vi "Begin.vi"(11 "Image Size":T3=enum."160x120") -> (0 "error out":errorcluster)   [LabVIEW 2012]
doc: "Called before other user functions, this VI is expected to open initial I/O refnums, load in file data, and do all program initialization. Notice that the <B>error out</B> terminal is simply used for data flow. Wiring it to other structures or subVIs ensures that this VI runs first."
uses:
  <vilib>/Rock Robotics/WPI/Camera/WPI_CameraImageSize.ctl
  <vilib>/Rock Robotics/SystemInterfaces/DIO/FPGA_DIOChannel.ctl
  <vilib>/Rock Robotics/SystemInterfaces/Typedef/FPGA_TypedefDigitalModule.ctl
  <vilib>/Rock Robotics/WPI/Joystick/WPI_JoystickDeviceEnum.ctl
  <vilib>/Rock Robotics/WPI/Camera/WPI_CameraWhite Balance Values.ctl
  <vilib>/Rock Robotics/WPI/Camera/WPI_CameraExposure Values.ctl
  <vilib>/Rock Robotics/WPI/Camera/WPI_CameraFrameRate.ctl
  <vilib>/Rock Robotics/SystemInterfaces/DIO/FPGA_DIOPWMChannel.ctl
  <vilib>/Rock Robotics/SystemInterfaces/AI/FPGA_AIChannel.ctl
  <vilib>/Rock Robotics/WPI/Encoder/WPI_EncoderType.ctl
  <vilib>/Rock Robotics/WPI/RobotDrive/WPI_RobotDriveOpen2MotorWithVictor.vi
  <vilib>/Rock Robotics/WPI/Counter/WPI_CounterDigitalInputToDigitalSource.vi
  <vilib>/Rock Robotics/WPI/MotorControl/WPI_MotorControlOpen Victor.vi
panel:
  in  "DIO Module 4":T1
  in  "B Channel 4":T2=enum."DIO 7"
  in  "A Channel 4":T2=enum."DIO 6"
  in  "DIO Module 3":T1
  in  "B Channel 3":T2=enum."DIO 5"
  in  "A Channel 3":T2=enum."DIO 4"
  in  "DIO Module 2":T1
  in  "B Channel 2":T2=enum."DIO 9"
  in  "A Channel 2":T2=enum."DIO 8"
  in  "DIO Module":T1
  in  "B Channel":T2=enum."DIO 12"
  in  "A Channel":T2=enum."DIO 11"
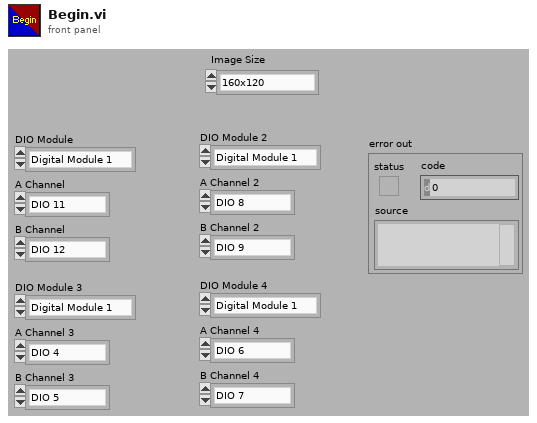
[diagram p1: front panel]
types:
  T1 = typedef "FPGA_TypedefDigitalModule.ctl" = enum16{"Digital Module 1", "Digital Module 2"}
  T2 = typedef "FPGA_DIOChannel.ctl" = enum8{"DIO 1", "DIO 2", "DIO 3", "DIO 4", "DIO 5", "DIO 6", "DIO 7", "DIO 8", "DIO 9", "DIO 10", "DIO 11", "DIO 12", "DIO 13", "DIO 14", "Invalid"}
  T3 = typedef "WPI_CameraImageSize.ctl" = enum16{"640x480", "320x240", "160x120"}
  T4 = typedef "WPI_EncoderType.ctl" = enum16{"1x", "2x", "4x"}
  T5 = typedef "FPGA_DIOPWMChannel.ctl" = enum8{"PWM 1", "PWM 2", "PWM 3", "PWM 4", "PWM 5", "PWM 6", "PWM 7", "PWM 8", "PWM 9", "PWM 10", "Invalid"}
  T6 = typedef "FPGA_AIChannel.ctl" = enum8{"AI 1", "AI 2", "AI 3", "AI 4", "AI 5", "AI 6", "AI 7", "AI 8", "Invalid"}
  T7 = typedef "WPI_CameraFrameRate.ctl" = u32
  T8 = typedef "WPI_CameraExposure Values.ctl" = enum16{"Auto", "Flicker-free 50 Hz", "Flicker-free 60 Hz", "Hold current"}
  T9 = typedef "WPI_CameraWhite Balance Values.ctl" = enum16{"Auto", "Fixed indoor", "Fixed outdoor 1", "Fixed outdoor 2", "Fixed fluorescent 1", "Fixed fluorescent 2", "Hold current"}
  T10 = typedef "WPI_JoystickDeviceEnum.ctl" = enum16{"USB 1", "USB 2", "USB 3", "USB 4", "Kinect 1", "Kinect 2"}
  T11 = typedef "WPI_DigitalInputDevRef.ctl" = cluster{"DevStatus":errorcluster, "DIO Channel":T2, "Digital Module":T1}
  T12 = typedef "FPGA_CounterEncoderSourceConvertionLVSourceType.ctl" = cluster{"DevStatus":errorcluster, "AnalogTriggerMode?":bool, "DigitalMode":cluster{"Digital Module":T1, "DIO Channel":T13}, "AnalogTriggerMode":cluster{"AnalogTriggerIndex":T14, "OutputType":T15}}
  T13 = typedef "FPGA_DIODigitalSourceChannel.ctl" = enum8{"DIO 1", "DIO 2", "DIO 3", "DIO 4", "DIO 5", "DIO 6", "DIO 7", "DIO 8", "DIO 9", "DIO 10", "DIO 11", "DIO 12", "DIO 13", "DIO 14", "Disabled"}
  T14 = typedef "FPGA_AnalogTriggerIndex.ctl" = enum8{"Trig 0", "Trig 1", "Trig 2", "Trig 3", "Trig 4", "Trig 5", "Trig 6", "Trig 7", "Invalid"}
  T15 = typedef "FPGA_AnalogTriggerOutType.ctl" = enum16{"InWindow", "TriggerState", "Rising", "Falling"}
  T16 = typedef "WPI_JoystickDevRef.ctl" = cluster{"Device":T10}
  T17 = typedef "WPI_CameraDevRef.ctl" = cluster{"Camera Address":string, "CameraStatus":errorcluster, "Acquire Image Notifier":refnum<notifier>}
  T18 = typedef "WPI_RobotDriveDevRef.ctl" = cluster{"DevStatus":errorcluster, "Motors[]":T19[], "Square Inputs":bool, "Max Output":dbl, "Isochronous":bool}
  T19 = typedef "WPI_MotorControlDeviceRef.ctl" = cluster{"DeviceStatus":errorcluster, "Type":enum16{"PWM", "CAN"}, "PWM":cluster{"Digital Module":T1, "PWM Channel":T5, "DeadBand":T20}, "CAN":cluster{"Device Number":u8, "Control Mode":T21, "Semaphore":T22, "Max Vout":dbl}, "Invert":bool, "TransformRef":T23, "InvTransformRef":T23}
  T20 = typedef "WPI_PWMDeadband.ctl" = cluster{"Name":string, "maxPositivePwm":i32, "minPositivePwm":i32, "centerPwm":i32, "maxNegativePwm":i32, "minNegativePwm":i32, "angularRange":u16}
  T21 = typedef "WPI_CANJaguar_ControlMode.ctl" = enum8{"Percent VBus", "Current", "Speed", "Position", "Voltage"}
  T22 = typedef "Semaphore RefNum" = refnum<k1>
  T23 = typedef "WPI_PWMTransform_ConPane.ctl" = refnum<vi>
  T24 = typedef "WPI_EncoderDevRef.ctl" = cluster{"DevStatus":errorcluster, "EncoderIndex":T25, "CounterIndex":T26, "DistancePerCount":dbl, "Decoding Type":T4}
  T25 = typedef "FPGA_EncoderIdx.ctl" = enum8{"Enc 0", "Enc 1", "Enc 2", "Enc 3", "Invalid"}
  T26 = typedef "FPGA_CounterCtrSystemIndex.ctl" = enum8{"Ctr 0", "Ctr 1", "Ctr 2", "Ctr 3", "Ctr 4", "Ctr 5", "Ctr 6", "Ctr 7", "Invalid"}
  T27 = typedef "WPI_AnalogChannelDevRef.ctl" = cluster{"DevStatus":errorcluster, "Analog Module":T28, "Analog Channel":T6}
  T28 = typedef "FPGA_TypedefAnalogModule.ctl" = enum16{"Analog Module 1", "Analog Module 2"}
  T29 = typedef "WPI_DigitalOutputDevRef.ctl" = cluster{"Digital Module":T1, "DIO Channel":T2, "DevStatus":errorcluster}
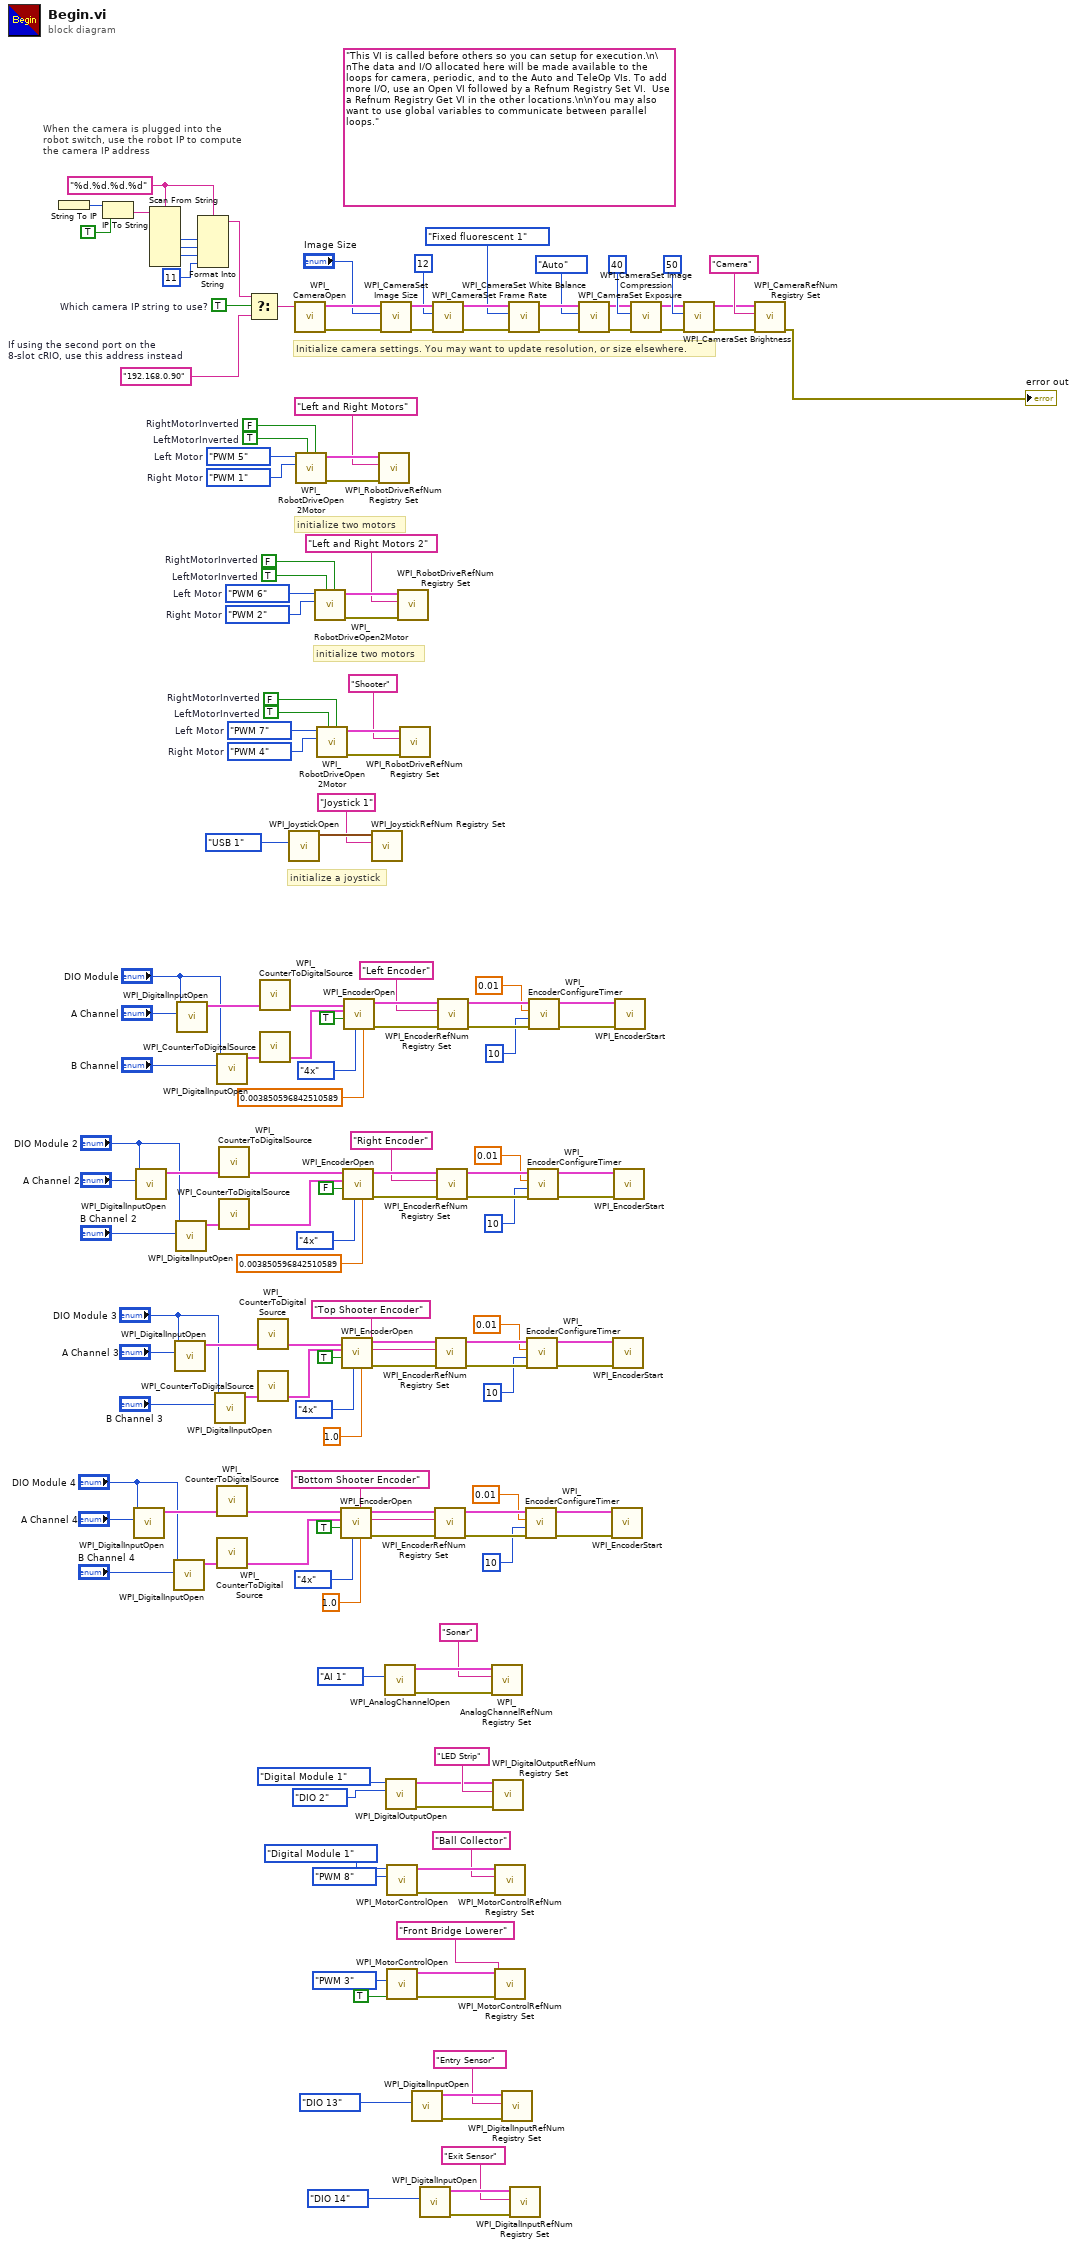
[diagram p0: block diagram]
diagram:
  w95 = FPGA_DIOPWMChannel."PWM 1"  # Right Motor
  w96 = FPGA_DIOPWMChannel."PWM 5"  # Left Motor
  w100 = TRUE  # LeftMotorInverted
  w101 = FALSE  # RightMotorInverted
  w102 = FPGA_DIOPWMChannel."PWM 2"  # Right Motor
  w103 = FPGA_DIOPWMChannel."PWM 6"  # Left Motor
  w107 = TRUE  # LeftMotorInverted
  w108 = FALSE  # RightMotorInverted
  w119 = FPGA_DIOPWMChannel."PWM 4"  # Right Motor
  w120 = FPGA_DIOPWMChannel."PWM 7"  # Left Motor
  w124 = TRUE  # LeftMotorInverted
  w125 = FALSE  # RightMotorInverted
  w126 = TRUE  # Which camera IP string to use?
  w130 = "%d.%d.%d.%d" ("format string")
  (unwired) "This VI is called before others so you can setup for execution.\n\nThe data and I/O allocated here will be made available to the loops for camera, periodic, and to the Auto and TeleOp VIs. To add more I/O, use an Open VI followed by a Refnum Registry Set VI.  Use a Refnum Registry Get VI in the other locations.\n\nYou may also want to use global variables to communicate between parallel loops."
  w127 = "192.168.0.90"  # If using the second port on the 8-slot cRIO, use this address instead
  # "initialize two motors"
  # "initialize two motors"
  # "When the camera is plugged into the\nrobot switch, use the robot IP to compute\nthe camera IP address"
  # "initialize a joystick"
  # "Initialize camera settings. You may want to update resolution, or size elsewhere."
  n1 = String To IP() -> (0:w137:u32)  [unwired: 1 in]
  n2 = IP To String(1:TRUE ("dot notation? (F)"), 2:w137) -> (0:w135:string)
  n3 = call <vilib>:"WPI_DigitalInputOpen.vi"("DIO Channel"="A Channel 4", "Digital Module (Module 1)"="DIO Module 4") -> ("DigitalInputDevRef"=w9:T11)  [unwired: 1 in, 8 out]
  n4 = call <vilib>:"WPI_DigitalInputOpen.vi"("DIO Channel"="A Channel 2", "Digital Module (Module 1)"="DIO Module 2") -> ("DigitalInputDevRef"=w69:T11)  [unwired: 1 in, 8 out]
  n5 = Scan From String(format string=w130, input string=w135) -> (output 1=w134:i32, output 2=w133:i32, output 3=w132:i32)  [unwired: 7 in, 3 out]
  n6 = call <vilib>:"WPI_DigitalInputOpen.vi"("DIO Channel"="B Channel 4", "Digital Module (Module 1)"="DIO Module 4") -> ("DigitalInputDevRef"=w10:T11)  [unwired: 1 in, 8 out]
  n7 = call <vilib>:"WPI_DigitalInputOpen.vi"("DIO Channel"="A Channel 3", "Digital Module (Module 1)"="DIO Module 3") -> ("DigitalInputDevRef"=w16:T11)  [unwired: 1 in, 8 out]
  n8 = call <vilib>:"WPI_DigitalInputOpen.vi"("DIO Channel"="B Channel 2", "Digital Module (Module 1)"="DIO Module 2") -> ("DigitalInputDevRef"=w70:T11)  [unwired: 1 in, 8 out]
  n9 = call <vilib>:"WPI_DigitalInputOpen.vi"("DIO Channel"="A Channel", "Digital Module (Module 1)"="DIO Module") -> ("DigitalInputDevRef"=w76:T11)  [unwired: 1 in, 8 out]
  n10 = Format Into String(format string=w130, w134, w133, w132, 11 ("Compression")) -> (resulting string=w128:string)  [unwired: 2 in, 1 out]
  n11 = call <vilib>:"WPI_DigitalInputOpen.vi"("DIO Channel"="B Channel 3", "Digital Module (Module 1)"="DIO Module 3") -> ("DigitalInputDevRef"=w17:T11)  [unwired: 1 in, 8 out]
  n12 = call <vilib>:"WPI_DigitalInputOpen.vi"("DIO Channel"="B Channel", "Digital Module (Module 1)"="DIO Module") -> ("DigitalInputDevRef"=w77:T11)  [unwired: 1 in, 8 out]
  n13 = call-poly <vilib>:"WPI_CounterToDigitalSource.vi"("DigitalInputDevRef"=w9) -> ("Digital Source"=w4:T12)  [unwired: 6 out]
  n14 = call-poly <vilib>:"WPI_CounterToDigitalSource.vi"("DigitalInputDevRef"=w10) -> ("Digital Source"=w5:T12)  [unwired: 6 out]
  n15 = call-poly <vilib>:"WPI_CounterToDigitalSource.vi"("DigitalInputDevRef"=w69) -> ("Digital Source"=w64:T12)  [unwired: 6 out]
  n16 = call-poly <vilib>:"WPI_CounterToDigitalSource.vi"("DigitalInputDevRef"=w70) -> ("Digital Source"=w65:T12)  [unwired: 6 out]
  n17 = Select(t=w128, s=w126, f=w127) -> (s? t:f=w129:string)
  n18 = call-poly <vilib>:"WPI_CounterToDigitalSource.vi"("DigitalInputDevRef"=w16) -> ("Digital Source"=w11:T12)  [unwired: 6 out]
  n19 = call-poly <vilib>:"WPI_CounterToDigitalSource.vi"("DigitalInputDevRef"=w17) -> ("Digital Source"=w12:T12)  [unwired: 6 out]
  n20 = call-poly <vilib>:"WPI_CounterToDigitalSource.vi"("DigitalInputDevRef"=w76) -> ("Digital Source"=w71:T12)  [unwired: 6 out]
  n21 = call-poly <vilib>:"WPI_CounterToDigitalSource.vi"("DigitalInputDevRef"=w77) -> ("Digital Source"=w72:T12)  [unwired: 6 out]
  n22 = call <vilib>:"WPI_JoystickOpen.vi"("JoystickDevice"=WPI_JoystickDeviceEnum."USB 1") -> ("JoystickDevRef"=w160:T16)  [unwired: 10 out]
  n23 = call <vilib>:"WPI_CameraOpen.vi"("Camera Address"=w129) -> ("error out"=w150:errorcluster, "CameraDevRef"=w151:T17)  [unwired: 2 in, 7 out]
  n24 = call-poly <vilib>:"WPI_RobotDriveOpen2Motor.vi"("Right Motor Inverted"=w101, "Left Motor Inverted"=w100, "Right Motor"=w95, "Left Motor"=w96) -> ("error out"=w97:errorcluster, "RobotDriveDevRef"=w99:T18)  [unwired: 1 in, 5 out]
  n25 = call-poly <vilib>:"WPI_RobotDriveOpen2Motor.vi"("Right Motor Inverted"=w108, "Left Motor Inverted"=w107, "Right Motor"=w102, "Left Motor"=w103) -> ("error out"=w104:errorcluster, "RobotDriveDevRef"=w106:T18)  [unwired: 1 in, 5 out]
  n26 = call-poly <vilib>:"WPI_RobotDriveOpen2Motor.vi"("Right Motor Inverted"=w125, "Left Motor Inverted"=w124, "Right Motor"=w119, "Left Motor"=w120) -> ("error out"=w121:errorcluster, "RobotDriveDevRef"=w123:T18)  [unwired: 1 in, 5 out]
  n27 = call <vilib>:"WPI_EncoderOpen.vi"("DistancePerCount"=1.0, "Decoding Type"=WPI_EncoderType."4x", "Invert Direction (False)"=TRUE, "BSource"=w5, "ASource"=w4) -> ("error out"=w25:errorcluster, "EncoderDevRef"=w26:T24)  [unwired: 5 in]
  n28 = call <vilib>:"WPI_EncoderOpen.vi"("DistancePerCount"=1.0, "Decoding Type"=WPI_EncoderType."4x", "Invert Direction (False)"=TRUE, "BSource"=w12, "ASource"=w11) -> ("error out"=w36:errorcluster, "EncoderDevRef"=w37:T24)  [unwired: 5 in]
  n29 = call <vilib>:"WPI_EncoderOpen.vi"("DistancePerCount"=0.003850596842510589, "Decoding Type"=WPI_EncoderType."4x", "Invert Direction (False)"=FALSE, "BSource"=w65, "ASource"=w64) -> ("error out"=w85:errorcluster, "EncoderDevRef"=w86:T24)  [unwired: 5 in]
  n30 = call <vilib>:"WPI_EncoderOpen.vi"("DistancePerCount"=0.003850596842510589, "Decoding Type"=WPI_EncoderType."4x", "Invert Direction (False)"=TRUE, "BSource"=w72, "ASource"=w71) -> ("error out"=w111:errorcluster, "EncoderDevRef"=w112:T24)  [unwired: 5 in]
  n31 = call <vilib>:"WPI_JoystickRefNum Registry Set.vi"("refnum name"="Joystick 1", "JoystickDevRef"=w160) -> ()  [unwired: 1 in, 9 out]
  n32 = call <vilib>:"WPI_RobotDriveRefNum Registry Set.vi"("error in (no error)"=w97, "refnum name"="Left and Right Motors", "RobotDriveDevRef"=w99) -> ()  [unwired: 9 out]
  n33 = call <vilib>:"WPI_CameraSet Image Size.vi"("error in (no error)"=w150, "Image Size"="Image Size", "CameraDevRef"=w151) -> ("error out"=w149:errorcluster, "CameraDevRef Out"=w152:T17)  [unwired: 7 out]
  n34 = call <vilib>:"WPI_AnalogChannelOpen.vi"("Analog Channel"=FPGA_AIChannel."AI 1") -> ("error out"=w116:errorcluster, "AIDeviceRef"=w118:T27)  [unwired: 9 in]
  n35 = call <vilib>:"WPI_DigitalOutputOpen.vi"("DIO Channel"=FPGA_DIOChannel."DIO 2", "Digital Module (Module 1)"=FPGA_TypedefDigitalModule."Digital Module 1") -> ("error out"=w44:errorcluster, "DigitalOutputDevRef"=w45:T29)  [unwired: 8 in]
  n36 = call-poly <vilib>:"WPI_MotorControlOpen.vi"("PWM Channel"=FPGA_DIOPWMChannel."PWM 8", "Digital Module (Module 1)"=FPGA_TypedefDigitalModule."Digital Module 1") -> ("error out"=w62:errorcluster, "MotorControlDeviceRef"=w61:T19)  [unwired: 8 in]
  n37 = call-poly <vilib>:"WPI_MotorControlOpen.vi"("Invert"=TRUE, "PWM Channel"=FPGA_DIOPWMChannel."PWM 3") -> ("error out"=w58:errorcluster, "MotorControlDeviceRef"=w57:T19)  [unwired: 8 in]
  n38 = call <vilib>:"WPI_RobotDriveRefNum Registry Set.vi"("error in (no error)"=w104, "refnum name"="Left and Right Motors 2", "RobotDriveDevRef"=w106) -> ()  [unwired: 9 out]
  n39 = call <vilib>:"WPI_RobotDriveRefNum Registry Set.vi"("error in (no error)"=w121, "refnum name"="Shooter", "RobotDriveDevRef"=w123) -> ()  [unwired: 9 out]
  n40 = call <vilib>:"WPI_DigitalInputOpen.vi"("DIO Channel"=FPGA_DIOChannel."DIO 13") -> ("error out"=w54:errorcluster, "DigitalInputDevRef"=w55:T11)  [unwired: 9 in]
  n41 = call <vilib>:"WPI_DigitalInputOpen.vi"("DIO Channel"=FPGA_DIOChannel."DIO 14") -> ("error out"=w50:errorcluster, "DigitalInputDevRef"=w51:T11)  [unwired: 9 in]
  n42 = call <vilib>:"WPI_CameraSet Frame Rate.vi"("error in (no error)"=w149, "Frame Rate (fps)"=T7 12, "CameraDevRef"=w152) -> ("error out"=w148:errorcluster, "CameraDevRef Out"=w154:T17)  [unwired: 7 out]
  n43 = call <vilib>:"WPI_EncoderRefNum Registry Set.vi"("error in (no error)"=w25, "refnum name"="Bottom Shooter Encoder", "EncoderDevRef"=w26) -> ("error out"=w21:errorcluster, "EncoderDevRef"=w23:T24)  [unwired: 7 in]
  n44 = call <vilib>:"WPI_EncoderRefNum Registry Set.vi"("error in (no error)"=w36, "refnum name"="Top Shooter Encoder", "EncoderDevRef"=w37) -> ("error out"=w32:errorcluster, "EncoderDevRef"=w34:T24)  [unwired: 7 in]
  n45 = call <vilib>:"WPI_EncoderRefNum Registry Set.vi"("error in (no error)"=w85, "refnum name"="Right Encoder", "EncoderDevRef"=w86) -> ("error out"=w81:errorcluster, "EncoderDevRef"=w83:T24)  [unwired: 7 in]
  n46 = call <vilib>:"WPI_EncoderRefNum Registry Set.vi"("error in (no error)"=w111, "refnum name"="Left Encoder", "EncoderDevRef"=w112) -> ("error out"=w92:errorcluster, "EncoderDevRef"=w94:T24)  [unwired: 7 in]
  n47 = call <vilib>:"WPI_AnalogChannelRefNum Registry Set.vi"("error in (no error)"=w116, "refnum name"="Sonar", "AIDeviceRef"=w118) -> ()  [unwired: 7 in, 2 out]
  n48 = call <vilib>:"WPI_DigitalOutputRefNum Registry Set.vi"("error in (no error)"=w44, "refnum name"="LED Strip", "DigitalOutputDevRef"=w45) -> ()  [unwired: 7 in, 2 out]
  n49 = call <vilib>:"WPI_MotorControlRefNum Registry Set.vi"("error in (no error)"=w62, "refnum name"="Ball Collector", "MotorControlDevRef"=w61) -> ()  [unwired: 7 in, 2 out]
  n50 = call <vilib>:"WPI_MotorControlRefNum Registry Set.vi"("error in (no error)"=w58, "refnum name"="Front Bridge Lowerer", "MotorControlDevRef"=w57) -> ()  [unwired: 7 in, 2 out]
  n51 = call <vilib>:"WPI_DigitalInputRefNum Registry Set.vi"("error in (no error)"=w54, "refnum name"="Entry Sensor", "DigitalInputDevRef"=w55) -> ()  [unwired: 7 in, 2 out]
  n52 = call <vilib>:"WPI_CameraSet White Balance.vi"("error in (no error)"=w148, "White Balance"=WPI_CameraWhite_Balance_Values."Fixed fluorescent 1", "CameraDevRef"=w154) -> ("error out"=w147:errorcluster, "CameraDevRef Out"=w153:T17)  [unwired: 7 out]
  n53 = call <vilib>:"WPI_DigitalInputRefNum Registry Set.vi"("error in (no error)"=w50, "refnum name"="Exit Sensor", "DigitalInputDevRef"=w51) -> ()  [unwired: 7 in, 2 out]
  n54 = call <vilib>:"WPI_EncoderConfigureTimer.vi"("error in (no error)"=w21, "Number Samples to Average"=u8 10, "Minimum Rate"=0.01, "EncoderDevRef"=w23) -> ("error out"=w20:errorcluster, "EncoderDevRef"=w22:T24)  [unwired: 6 in]
  n55 = call <vilib>:"WPI_EncoderConfigureTimer.vi"("error in (no error)"=w32, "Number Samples to Average"=u8 10, "Minimum Rate"=0.01, "EncoderDevRef"=w34) -> ("error out"=w31:errorcluster, "EncoderDevRef"=w33:T24)  [unwired: 6 in]
  n56 = call <vilib>:"WPI_EncoderConfigureTimer.vi"("error in (no error)"=w81, "Number Samples to Average"=u8 10, "Minimum Rate"=0.01, "EncoderDevRef"=w83) -> ("error out"=w80:errorcluster, "EncoderDevRef"=w82:T24)  [unwired: 6 in]
  n57 = call <vilib>:"WPI_EncoderConfigureTimer.vi"("error in (no error)"=w92, "Number Samples to Average"=u8 10, "Minimum Rate"=0.01, "EncoderDevRef"=w94) -> ("error out"=w91:errorcluster, "EncoderDevRef"=w93:T24)  [unwired: 6 in]
  n58 = call <vilib>:"WPI_CameraSet Exposure.vi"("error in (no error)"=w147, "Exposure"=WPI_CameraExposure_Values."Auto", "CameraDevRef"=w153) -> ("error out"=w146:errorcluster, "CameraDevRef Out"=w156:T17)  [unwired: 7 out]
  n59 = call <vilib>:"WPI_EncoderStart.vi"("error in (no error)"=w20, "EncoderDevRef"=w22) -> ()  [unwired: 8 in, 2 out]
  n60 = call <vilib>:"WPI_EncoderStart.vi"("error in (no error)"=w31, "EncoderDevRef"=w33) -> ()  [unwired: 8 in, 2 out]
  n61 = call <vilib>:"WPI_EncoderStart.vi"("error in (no error)"=w80, "EncoderDevRef"=w82) -> ()  [unwired: 8 in, 2 out]
  n62 = call <vilib>:"WPI_EncoderStart.vi"("error in (no error)"=w91, "EncoderDevRef"=w93) -> ()  [unwired: 8 in, 2 out]
  n63 = call <vilib>:"WPI_CameraSet Image Compression.vi"("error in (no error)"=w146, "Compression"=40, "CameraDevRef"=w156) -> ("error out"=w145:errorcluster, "CameraDevRef Out"=w155:T17)  [unwired: 7 out]
  n64 = call <vilib>:"WPI_CameraSet Brightness.vi"("error in (no error)"=w145, "Brightness"=50, "CameraDevRef"=w155) -> ("error out"=w143:errorcluster, "CameraDevRef Out"=w144:T17)  [unwired: 7 out]
  n65 = call <vilib>:"WPI_CameraRefNum Registry Set.vi"("error in (no error)"=w143, "refnum name"="Camera", "CameraDevRef"=w144) -> ("error out"=→"error out":errorcluster)  [unwired: 8 out]
